vi "System Language.vi"() -> (3 "s? t:f":string)   [LabVIEW 2017]
uses:
  Communicable State Machine.lvlib
panel:
  out "Array of Strings":string[](array[string])
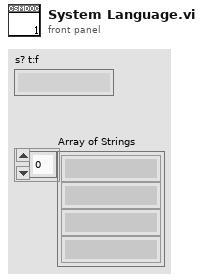
[diagram p1: front panel]
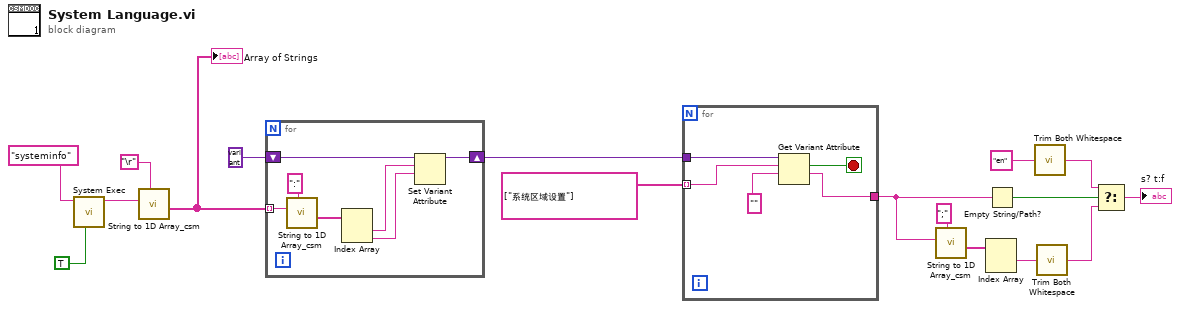
[diagram p0: block diagram]
diagram:
  n1 = call <vilib>:"System Exec.vi"("run minimized? (F)"=TRUE, "command line"="systeminfo") -> ("standard output"=w15:string)  [unwired: 6 in, 3 out]
  n2 = call "String to 1D Array_csm.vi"("delimiter (Tab)"="\r", "string"=w15) -> ("Array of Strings"=w13:string[])  [unwired: 9 in]
  "Array of Strings" <- w13
  n3 = for {
    tunnel: w13 -> [w24] mode=indexing
    shift-right: [w21] -> w11
    shift-left: variant -> [w22]
    n4 = call "String to 1D Array_csm.vi"("delimiter (Tab)"=":", "string"=w24) -> ("Array of Strings"=w20:string[])  [unwired: 9 in]
    n5 = Index Array(array=w20) -> (element #1=w19:string, element #2=w18:string)  [unwired: 2 in]
    n6 = Set Variant Attribute(Variant=w22, name=w19, value=w18) -> (Variant out=w21:variant)  [unwired: 1 in, 2 out]
  }
  n7 = for {
    tunnel: w11 -> [w29]
    tunnel: string[] ["系统区域设置"] ("name") -> [w28] mode=indexing
    tunnel: [w25] -> w5
    stop <- w27 stop-if-true
    n8 = Get Variant Attribute(Variant=w29, name=w28, default value (empty Variant)="" ("name")) -> (found=w27:bool, value=w25:string)  [unwired: 1 in, 2 out]
  }
  n9 = call "String to 1D Array_csm.vi"("delimiter (Tab)"=";", "string"=w5) -> ("Array of Strings"=w4:string[])  [unwired: 9 in]
  n10 = Index Array(array=w4) -> (element #1=w3:string)  [unwired: 2 in, 1 out]
  n11 = Empty String/Path?(string/path=w5) -> (empty?=w9:bool)
  n12 = call "Trim Both Whitespace.vi"("string"="en" ("f")) -> ("trimmed string"=w2:string)  [unwired: 1 in]
  n13 = call "Trim Both Whitespace.vi"("string"=w3) -> ("trimmed string"=w1:string)  [unwired: 1 in]
  n14 = Select(t=w2, s=w9, f=w1) -> (s? t:f=→"s? t:f":string)
